vi "Compute Distance.vi"(11 "Bounding Box":T1) -> (0 "Center":bool, 1 "Right":bool, 2 "Target Center (-1 to 1)":cluster{"X":dbl, "Y":dbl}, 3 "Distance (ft)":dbl, 4 "Left":bool, 5 "-1 to 1 Center of Target Adjusted":dbl)   [LabVIEW 2011]
doc: "Using the camera lens information and the real world width of the target, determine the distance to the target."
panel:
  out "+/- Outer Deadband":dbl
  in  "PixelsDeadbandInside":dbl=4.0
  out "RelativePixelCenter":dbl
  in  "PixelsDeadbandOverall":dbl=10.0
  in  "PixelsOffset":dbl=25.0
  in  "Y Image Resolution":i32=240
  in  "Camera view angle":dbl[](array[numeric])=[48.0, 43.5]
  in  "X Image Resolution":i32=320
  in  "Camera Type":enum16{"206", "1011"}(ring)=enum."1011"
  # "Actually 20, 10 on each side"
  # "Inner 8 pixels on each side"
  # "Axis 206\nAxis M1011"
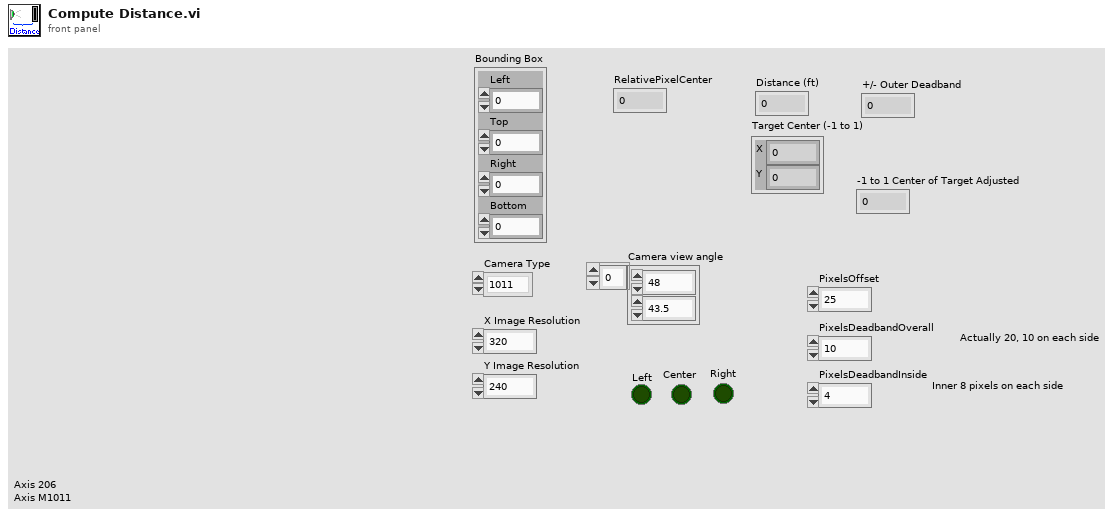
[diagram p1: front panel]
types:
  T1 = cluster{"Left":dbl, "Top":dbl, "Right":dbl, "Bottom":dbl}
  T2 = cluster{"X Image Resolution":i32, "Y Image Resolution":i32}
  T3 = cluster{"X Image Resolution":dbl, "Y Image Resolution":dbl}
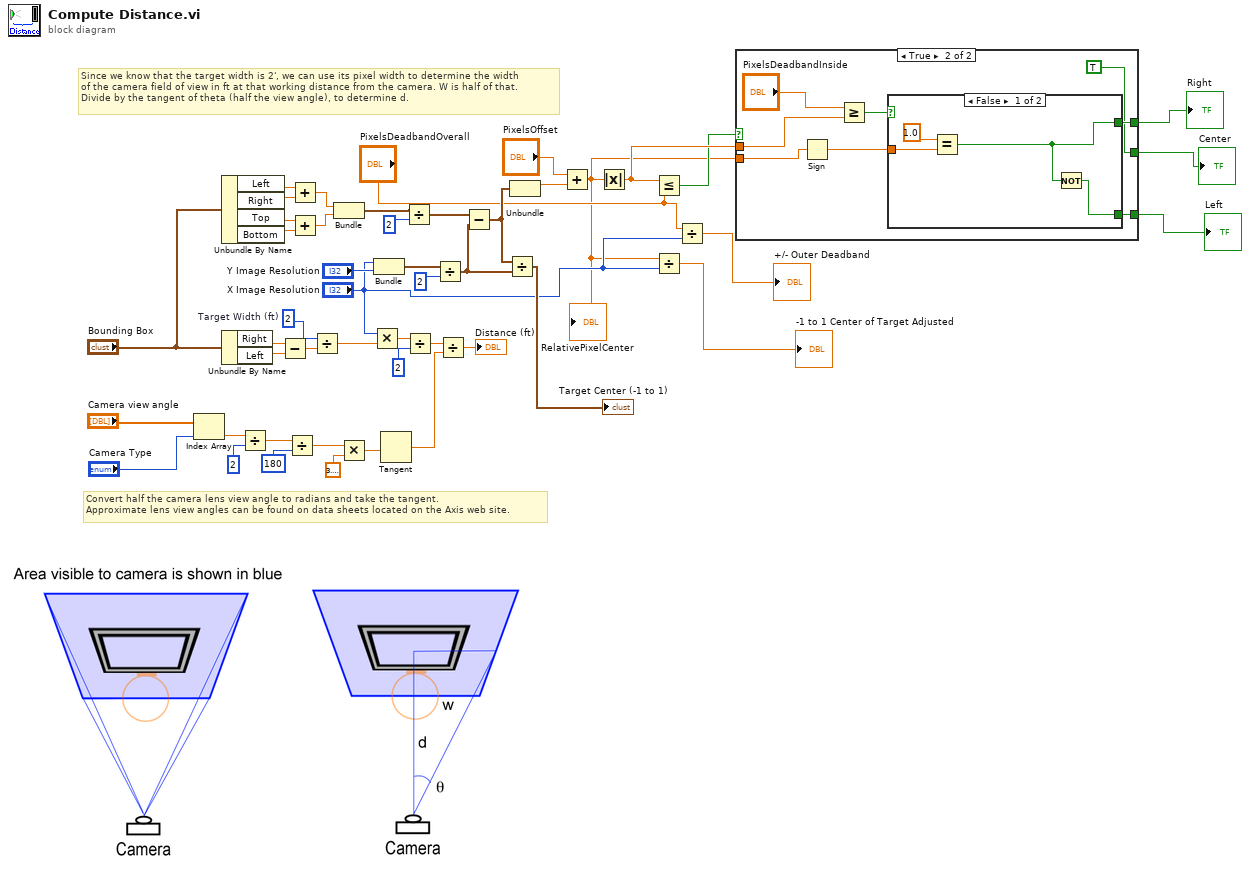
[diagram p0: block diagram]
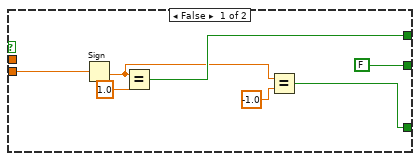
[diagram p2: hidden frame]
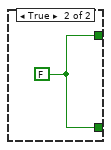
[diagram p3: hidden frame]
diagram:
  w30 = 2  # Target Width (ft)
  # "Convert half the camera lens view angle to radians and take the tangent.\nApproximate lens view angles can be found on data sheets located on the Axis web site."
  # "Since we know that the target width is 2', we can use its pixel width to determine the width\nof the camera field of view in ft at that working distance from the camera. W is half of that.\nDivide by the tangent of theta (half the view angle), to determine d."
  n1 = Index Array(array="Camera view angle", index="Camera Type") -> (element=w43:dbl)
  n2 = Unbundle By Name("Bounding Box") -> ("Left"=w25:dbl, "Right"=w26:dbl, "Top"=w28:dbl, "Bottom"=w27:dbl)
  n3 = Unbundle By Name("Bounding Box") -> ("Right"=w34:dbl, "Left"=w33:dbl)
  n4 = Divide(x=w43, y=2) -> (x/y=w40:dbl)
  n5 = Subtract(x=w34, y=w33) -> (x-y=w32:dbl)
  n6 = Divide(x=w40, y=180) -> (x/y=w39:dbl)
  n7 = Add(x=w25, y=w26) -> (x+y=w23:dbl)
  n8 = Add(x=w28, y=w27) -> (x+y=w22:dbl)
  n9 = Divide(x=w30, y=w32) -> (x/y=w31:dbl)
  n10 = Bundle(w23, w22) -> (w20:cluster{dbl, dbl})  [unwired: 1 in]
  n11 = Multiply(x=w39, y=3.141592653589793) -> (x*y=w41:dbl)
  n12 = Multiply(x="X Image Resolution", y=w31) -> (x*y=w35:dbl)
  n13 = Bundle("X Image Resolution"="X Image Resolution", "Y Image Resolution"="Y Image Resolution") -> (w16:T2)  [unwired: 1 in]
  n14 = Tangent(1:w41) -> (0:w47:dbl)
  n15 = Divide(x=w20, y=2) -> (x/y=w17:cluster{dbl, dbl})
  n16 = Divide(x=w35, y=2) -> (x/y=w37:dbl)
  n17 = Divide(x=w16, y=2) -> (x/y=w19:T3)
  n18 = Divide(x=w37, y=w47) -> (x/y=→"Distance (ft)":dbl)
  n19 = Subtract(x=w17, y=w19) -> (x-y=w15:cluster{dbl, dbl})
  n20 = Divide(x=w15, y=w19) -> (x/y=→"Target Center (-1 to 1)":cluster{dbl, dbl})
  n21 = Unbundle(w15) -> (w14:dbl)  [unwired: 1 out]
  n22 = Add(x="PixelsOffset", y=w14) -> (x+y=w2:dbl)
  "RelativePixelCenter" <- w2
  n23 = Absolute Value(x=w2) -> (abs(x)=w9:dbl)
  n24 = Less Or Equal?(x=w9, y="PixelsDeadbandOverall") -> (x <= y?=w8:bool)
  n25 = Divide(x=w2, y="X Image Resolution") -> (x/y=→"-1 to 1 Center of Target Adjusted":dbl)
  n26 = Divide(x="PixelsDeadbandOverall", y="X Image Resolution") -> (x/y=→"+/- Outer Deadband":dbl)
  n27 = case shown="True" w8 {
    tunnel: [w51 w60] -> w11
    tunnel: [FALSE TRUE] -> w12
    tunnel: [w48 w59] -> w10
    tunnel: w9 -> [_ w62]
    tunnel: w2 -> [w53 w58]
    frame False {
      n28 = Sign(1:w53) -> (0:w49:dbl)
      n29 = Equal?(x=w49, y=1.0) -> (x = y?=w51:bool)
      n30 = Equal?(x=w49, y=-1.0) -> (x = y?=w48:bool)
    }
    frame True {
      n31 = Sign(1:w58) -> (0:w57:dbl)
      n32 = Greater Or Equal?(x="PixelsDeadbandInside", y=w62) -> (x >= y?=w61:bool)
      n33 = case shown="False" w61 {
        tunnel: [w64 w67] -> w60
        tunnel: [w63 w67] -> w59
        tunnel: w57 -> [w66 _]
        frame False {
          n34 = Equal?(x=1.0, y=w66) -> (x = y?=w64:bool)
          n35 = Not(x=w64) -> (.not. x?=w63:bool)
        }
        frame True {
          w67 = FALSE
        }
      }
    }
  }
  "Center" <- w12
  "Left" <- w10
  "Right" <- w11
